vi "SM motor tw.vi"(0 "SM Config":T3={"VISA Serial ref"="COM3", "Motor Config"={"DriveRatio (mm/rev)"=10.16, "PosLimit + (mm)"=200.0, "PosLimit - (mm)"=0.0, "EncoderRatio (count/rev)"=2000.0, "MotorType"=enum."SM17"}} {"Motor Config"."EncoderRatio (count/rev)" format="%.2f"; "Motor Config"."PosLimit - (mm)" format="%.3f"; "Motor Config"."PosLimit + (mm)" format="%.3f"; "Motor Config"."DriveRatio (mm/rev)" format="%.2f"}, 1 "SM setting":T2={"Acceleration (mm/sec^2)"=1000.0, "Velocity (mm/sec)"=1.0, "Position (mm)"=0.0} {"Position (mm)" format="%.3f"; "Velocity (mm/sec)" format="%.3f"; "Acceleration (mm/sec^2)" format="%.3f"}, 2 "Move":bool, 3 "Stop motion":bool) -> (7 "Status":T1, 8 "Position (mm)":dbl)   [LabVIEW 2015]
uses:
  magnetometers/smi/labview/CPM20Software/SmartMotor.llb/SM Config.ctl
  magnetometers/smi/labview/CPM20Software/SmartMotor.llb/SM MotorConfig.ctl
  magnetometers/smi/labview/CPM20Software/SmartMotor.llb/SM Status.ctl
  magnetometers/smi/labview/CPM20Software/SmartMotor.llb/SM SetAccel (mm/sec^2).vi
  magnetometers/smi/labview/CPM20Software/SmartMotor.llb/SM SetVelocity (mm/sec).vi
panel:
  out "error out":errorcluster
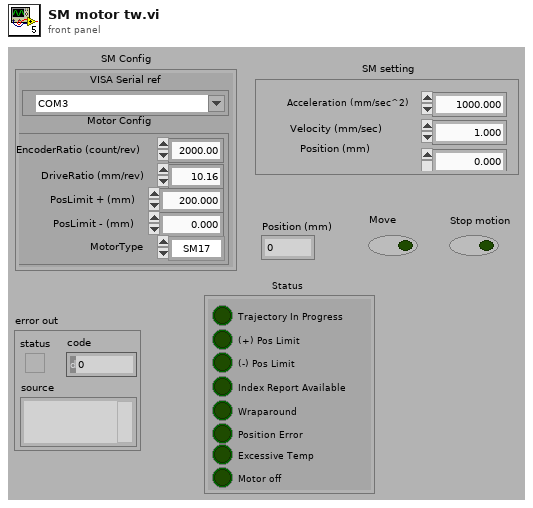
[diagram p1: front panel]
types:
  T1 = typedef "SM Status.ctl" = cluster{"Trajectory In Progress":bool, "(+) Pos Limit":bool, "(-) Pos Limit":bool, "Index Report Available":bool, "Wraparound":bool, "Position Error":bool, "Excessive Temp":bool, "Motor off":bool}
  T2 = cluster{"Acceleration (mm/sec^2)":dbl, "Velocity (mm/sec)":dbl, "Position (mm)":dbl}
  T3 = typedef "SM Config.ctl" = cluster{"VISA Serial ref":refnum<visa-resource-name>, "Motor Config":T4}
  T4 = typedef "SM MotorConfig.ctl" = cluster{"DriveRatio (mm/rev)":dbl, "PosLimit + (mm)":dbl, "PosLimit - (mm)":dbl, "EncoderRatio (count/rev)":dbl, "MotorType":enum16{"SM17", "SM23", "SM34", "SM42", "SM56"}}
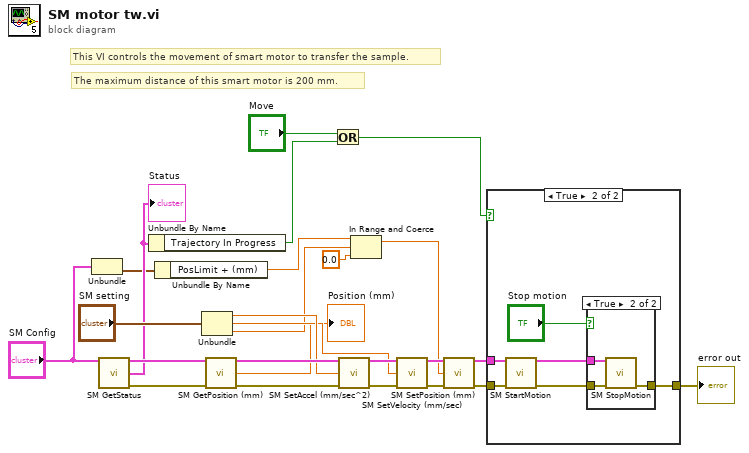
[diagram p0: block diagram]
diagram:
  # "The maximum distance of this smart motor is 200 mm."
  # "This VI controls the movement of smart motor to transfer the sample."
  n1 = Unbundle("SM Config") -> ("Motor Config"=w2:T4)  [unwired: 1 out]
  n2 = call "SM GetStatus.vi"("SM Config"="SM Config") -> ("SM Config dup"=w12:T3, "Status"=w10:T1, "error out"=w11:errorcluster)  [unwired: 1 in, 11 out]
  "Status" <- w10
  n3 = Unbundle By Name(w10) -> ("Trajectory In Progress"=w8:bool)
  n4 = Unbundle By Name(w2) -> ("PosLimit + (mm)"=w1:dbl)
  n5 = Unbundle("SM setting") -> ("Acceleration (mm/sec^2)"=w19:dbl, "Velocity (mm/sec)"=w18:dbl, "Position (mm)"=w5:dbl)
  n6 = call "SM GetPosition (mm).vi"("SM Config"=w12, "error in (no error)"=w11) -> ("SM Config dup"=w23:T3, "Axis Position (mm)"=→"Position (mm)":dbl, "error out"=w17:errorcluster)  [unwired: 11 out]
  n7 = Or(x="Move", y=w8) -> (x .or. y?=w7:bool)
  n8 = call "SM SetAccel (mm/sec^2).vi"("SM Config"=w23, "Acceleration (mm/sec^2)"=w19, "error in (no error)"=w17) -> ("SM Config dup"=w22:T3, "error out"=w16:errorcluster)  [unwired: 11 out]
  n9 = In Range and Coerce(upper limit=w1, x=w5, lower limit=0.0) -> (coerced(x)=w13:dbl)  [unwired: 1 out]
  n10 = call "SM SetVelocity (mm/sec).vi"("SM Config"=w22, "Velocity (mm/sec)"=w18, "error in (no error)"=w16) -> ("SM Config dup"=w21:T3, "error out"=w15:errorcluster)  [unwired: 11 out]
  n11 = call "SM SetPosition (mm).vi"("SM Config"=w21, "Position (mm)"=w13, "error in (no error)"=w15) -> ("SM Config dup"=w20:T3, "error out"=w14:errorcluster)  [unwired: 11 out]
  n12 = case shown="True" w7 {
    tunnel: w20 -> [_ w32]
    tunnel: w14 -> [w26 w31]
    tunnel: [w26 w27] -> w25
    frame False {
    }
    frame True {
      n13 = call "SM StartMotion.vi"("SM Config"=w32, "error in (no error)"=w31) -> ("SM Config dup"=w29:T3, "error out"=w28:errorcluster)  [unwired: 12 out]
      n14 = case shown="True" "Stop motion" {
        tunnel: w29 -> [_ w36]
        tunnel: w28 -> [w33 w35]
        tunnel: [w33 w34] -> w27
        frame False {
        }
        frame True {
          n15 = call "SM StopMotion.vi"("SM Config"=w36, "error in (no error)"=w35) -> ("error out"=w34:errorcluster)  [unwired: 1 in, 12 out]
        }
      }
    }
  }
  "error out" <- w25
